vi "GeneradosNoLineal.vi"(3 "Duración de los ceros":dbl=5.0, 4 "Duración de ciclo (s)":dbl=20.0, 5 "Periodo de muestreo":dbl=0.05) -> (0 "Numero de muestras":i32, 1 "Waveform Graph 2":waveform(dbl)(graph), 2 "Señal No linealidad":dbl[](array[numeric]))   [LabVIEW 2013]
uses:
  <vilib>/measure/NI_MABase.lvlib
panel:
  out "Waveform Graph":waveform(dbl)(graph)
  out "Y":dbl[](array[numeric])
  out "s":dbl
  out "Fs":dbl
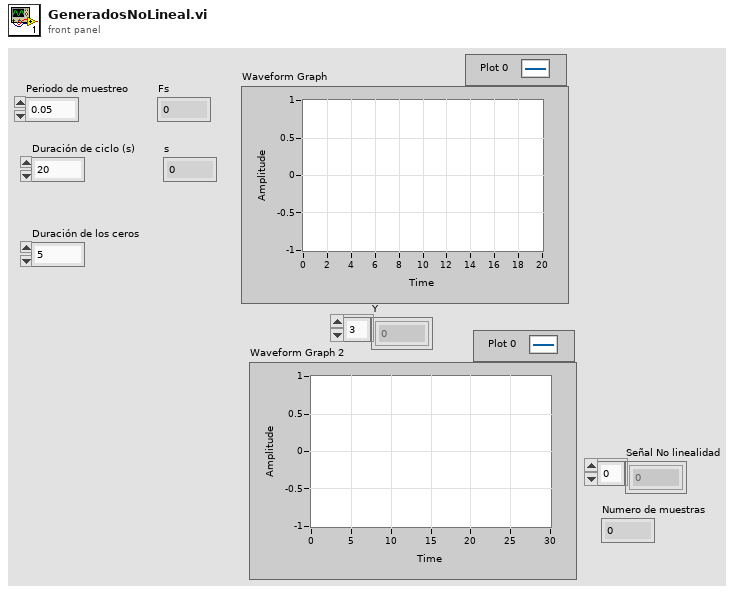
[diagram p1: front panel]
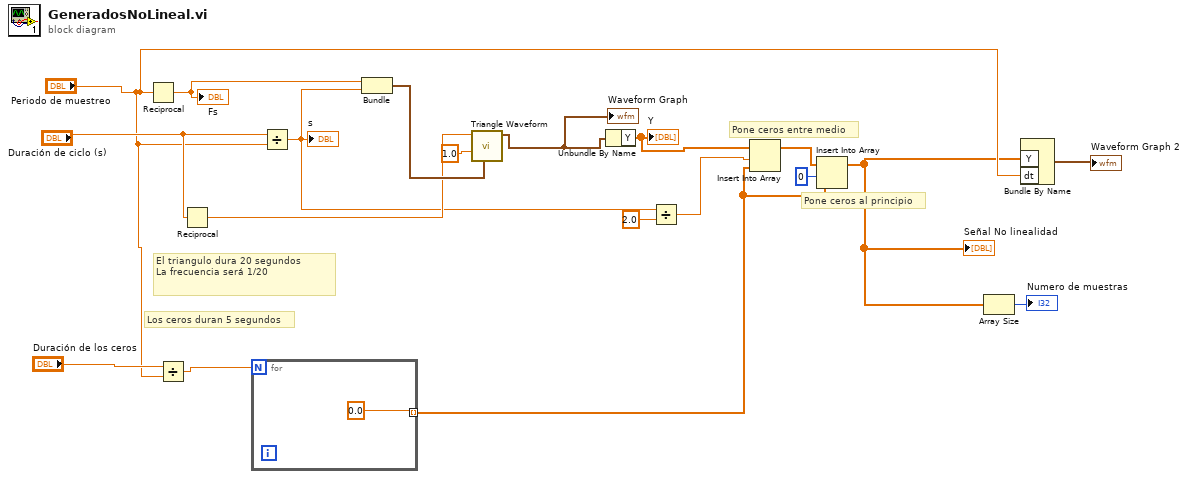
[diagram p0: block diagram]
diagram:
  # "Pone ceros al principio"
  # "Pone ceros entre medio"
  # "Los ceros duran 5 segundos"
  # "El triangulo dura 20 segundos\nLa frecuencia será 1/20"
  n1 = Reciprocal(x="Periodo de muestreo") -> (1/x=w16:dbl)
  "Fs" <- w16
  n2 = Divide(x="Duración de los ceros", y="Periodo de muestreo") -> (x/y=w8:dbl)
  n3 = Reciprocal(x="Duración de ciclo (s)") -> (1/x=w15:dbl)
  n4 = for {
    N: w8 -> [_]
    tunnel: [0.0] -> w3 mode=indexing
  }
  n5 = Divide(x="Duración de ciclo (s)", y="Periodo de muestreo") -> (x/y=w13:dbl)
  "s" <- w13
  n6 = Bundle(w16, w13) -> (w17:cluster{dbl, dbl})  [unwired: 1 in]
  n7 = call <vilib>:"Triangle Waveform.vi"("sampling info"=w17, "amplitude"=1.0, "frequency"=w15) -> ("signal out"=w18:waveform(dbl))  [unwired: 7 in, 1 out]
  "Waveform Graph" <- w18
  n8 = Unbundle By Name(w18) -> ("Y"=w11:dbl[])
  "Y" <- w11
  n9 = Divide(x=w13, y=2.0) -> (x/y=w10:dbl)
  n10 = Insert Into Array(array=w11, index=w10, new element=w3) -> (w2:dbl[])
  n11 = Insert Into Array(array=w2, index=0, new element=w3) -> (w1:dbl[])
  "Señal No linealidad" <- w1
  n12 = Array Size(array=w1) -> (size(s)=→"Numero de muestras":i32)
  n13 = Bundle By Name("Y"=w1, "dt"="Periodo de muestreo") -> (→"Waveform Graph 2":waveform(dbl))  [unwired: 1 in]
